vi "DispenseAtFixedPressTimePos.vi"() -> ()   [LabVIEW 2019]
uses:
  Other Models/EFD Ultimus V/EFD Ultimus V.lvlib
panel:
  in  "Calc":bool
  in  "DefaultPressure":dbl[](array[numeric])=[30.0, 21.0, 32.0, 22.0]
  out "PressureWillBeSetTo":dbl[](array[numeric])
  in  "error in (no error)":errorcluster
  out "AmtDispensed(g)":dbl
  out "CorrectionFactor":dbl=1.0
  in  "WtFor50Psi30Sec":dbl=1.039
  in  "PaperWtWithGlue(g)":dbl
  in  "PaperWt(g)":dbl
  out "TimeCalculated":dbl
  out "error out":errorcluster
  in  "Serial Configuration":T1={"Baud Rate "=115200, "Parity "=0, "Data Bits "=8, "Stop Bits"=10} {"Stop Bits" items=["1.0"=10, "1.5"=15, "2.0"=20]; "Data Bits" items=["7"=7, "8"=8]; "Parity" items=["None", "Odd", "Even"]; "Baud Rate" items=["9600"=9600, "19200"=19200, "38400"=38400, "115200"=115200]}
  in  "VISA resource name":refnum<visa-resource-name>="COM5"
  in  "Time(s)":dbl=30.0
  in  "PressureSet":dbl=50.0
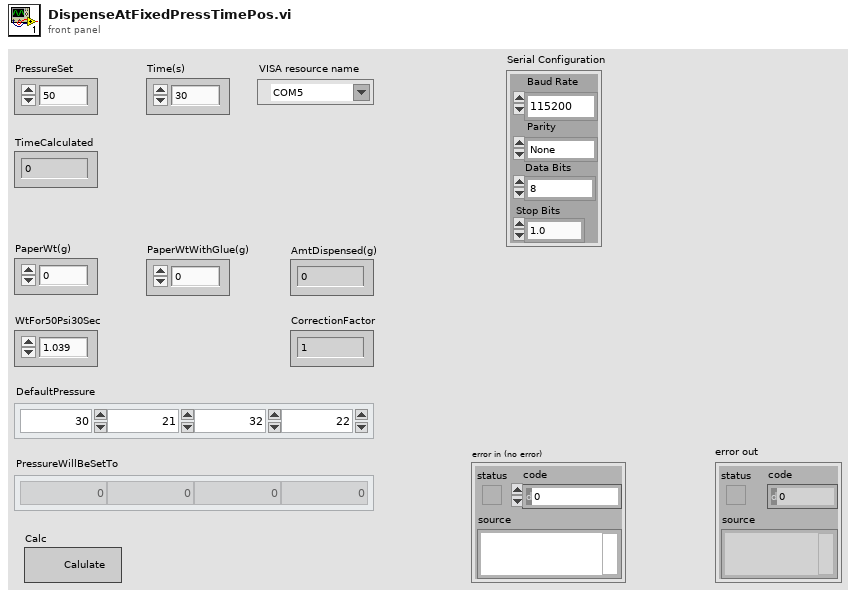
[diagram p1: front panel]
types:
  T1 = cluster{"Baud Rate ":u32, "Parity ":u16, "Data Bits ":u16, "Stop Bits":u16}
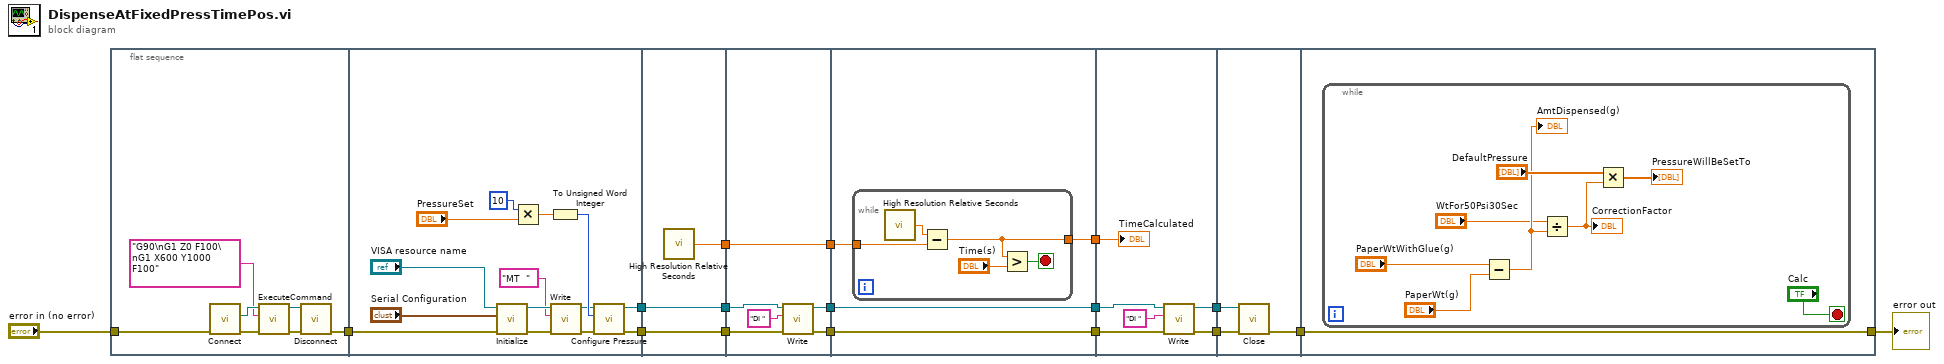
[diagram p0: block diagram]
diagram:
  n1 = flat-sequence {
    tunnel: "error in (no error)" -> [w19]
    tunnel: [w18] -> w2
    tunnel: [w26] -> w16
    tunnel: [w27] -> w15
    tunnel: w2 -> [w25]
    tunnel: [w41] -> w14
    tunnel: [w40] -> w13
    tunnel: [w39] -> w12
    tunnel: w16 -> [w41]
    tunnel: w15 -> [w40]
    tunnel: [w45] -> w11
    tunnel: [w44] -> w10
    tunnel: w14 -> [w47]
    tunnel: w13 -> [w46]
    tunnel: [w42] -> w9
    tunnel: w12 -> [w42]
    tunnel: w11 -> [w51]
    tunnel: w10 -> [w50]
    tunnel: [w51] -> w8
    tunnel: [w50] -> w7
    tunnel: w9 -> [w49]
    tunnel: [w48] -> w6
    tunnel: w8 -> [w61]
    tunnel: w7 -> [w62]
    tunnel: w6 -> [w57]
    tunnel: [w60] -> w5
    tunnel: [w59] -> w4
    tunnel: w5 -> [w65]
    tunnel: w4 -> [w64]
    tunnel: [w63] -> w1
    tunnel: [w66] -> w17
    tunnel: w1 -> [w66]
    frame #0 {
      n2 = call "Connect.vi"("error in (no error)"=w19) -> ("error out"=w23:errorcluster, "controller"=w24:refnum<k24>)  [unwired: 9 in]
      n3 = call "ExecuteCommand.vi"("error in (no error)"=w23, "Command Code"="G90\nG1 Z0 F100\nG1 X600 Y1000 F100", "controller in"=w24) -> ("error out"=w21:errorcluster, "controller out"=w22:refnum<k24>)  [unwired: 6 in, 1 out]
      n4 = call "Disconnect.vi"("error in (no error)"=w21, "controller"=w22) -> ("error out"=w18:errorcluster)  [unwired: 9 in]
    }
    frame #1 {
      n5 = call "Initialize.vi"("error in (no error)"=w25, "Serial Configuration"="Serial Configuration", "VISA resource name"="VISA resource name") -> ("error out"=w33:errorcluster, "VISA resource name out"=w32:refnum<visa-resource-name>)  [unwired: 7 in]
      n6 = Multiply(x=10, y="PressureSet") -> (x*y=w35:dbl)
      n7 = To Unsigned Word Integer(number=w35) -> (unsigned 16bit integer=w36:u16)
      n8 = call "Write.vi"("error in (no error)"=w33, "Command To Write"="MT  ", "VISA resource name"=w32) -> ("error out"=w37:errorcluster, "VISA resource name out"=w34:refnum<visa-resource-name>)  [unwired: 7 in]
      n9 = call "Configure Pressure.vi"("error in (no error)"=w37, "Pressure Setting (0000)"=w36, "VISA resource name"=w34) -> ("error out"=w27:errorcluster, "VISA resource name out"=w26:refnum<visa-resource-name>)  [unwired: 7 in]
    }
    frame #2 {
      n10 = call <vilib>:"High Resolution Relative Seconds.vi"() -> ("relative seconds"=w39:dbl)
    }
    frame #3 {
      n11 = call "Write.vi"("error in (no error)"=w46, "Command To Write"="DI ", "VISA resource name"=w47) -> ("error out"=w44:errorcluster, "VISA resource name out"=w45:refnum<visa-resource-name>)  [unwired: 7 in]
    }
    frame #4 {
      n12 = while {
        tunnel: w49 -> [w55]
        tunnel: [w52] -> w48
        stop <- w54 stop-if-true
        n13 = call <vilib>:"High Resolution Relative Seconds.vi"() -> ("relative seconds"=w56:dbl)
        n14 = Subtract(x=w56, y=w55) -> (x-y=w52:dbl)
        n15 = Greater?(x=w52, y="Time(s)") -> (0:w54:bool)
      }
    }
    frame #5 {
      n16 = call "Write.vi"("error in (no error)"=w62, "Command To Write"="DI ", "VISA resource name"=w61) -> ("error out"=w60:errorcluster, "VISA resource name out"=w59:refnum<visa-resource-name>)  [unwired: 7 in]
      "TimeCalculated" <- w57
    }
    frame #6 {
      n17 = call "Close.vi"("error in (no error)"=w65, "VISA resource name"=w64) -> ("error out"=w63:errorcluster)  [unwired: 9 in]
    }
    frame #7 {
      n18 = while {
        stop <- "Calc" stop-if-true
        n19 = Subtract(x="PaperWtWithGlue(g)", y="PaperWt(g)") -> (x-y=w70:dbl)
        "AmtDispensed(g)" <- w70
        n20 = Divide(x="WtFor50Psi30Sec", y=w70) -> (x/y=w68:dbl)
        "CorrectionFactor" <- w68
        n21 = Multiply(x="DefaultPressure", y=w68) -> (x*y=→"PressureWillBeSetTo":dbl[])
      }
    }
  }
  "error out" <- w17
